vi "16BitsTo4ByteFloat.vi"(9 "Array":bool[](array[boolean]), 10 "Array 2":bool[](array[boolean]), 11 "Sign":bool) -> (1 "Mantissa 2":dbl=1.4518749713897705 format="%.8f", 2 "Numeric":sgl, 3 "Exponent":i32=6)   [LabVIEW 2014]
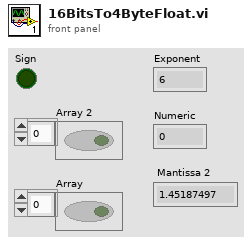
[diagram p1: front panel]
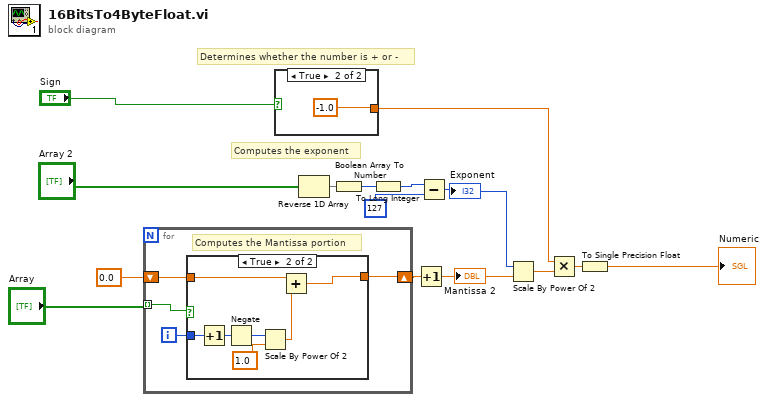
[diagram p0: block diagram]
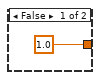
[diagram p2: hidden frame]
diagram:
  # "Computes the exponent"
  # "Determines whether the number is + or -"
  n1 = for {
    tunnel: "Array" -> [w19] mode=indexing
    shift-right: [w16] -> w2
    shift-left: 0.0 -> [w17]
    i -> [w18]
    # "Computes the Mantissa portion"
    n2 = case shown="True" w19 {
      tunnel: w18 -> [_ w27]
      tunnel: w17 -> [w20 w23]
      tunnel: [w20 w21] -> w16
      frame False {
      }
      frame True {
        n3 = Increment(x=w27) -> (x+1=w26:i32)
        n4 = Negate(x=w26) -> (-x=w25:i32)
        n5 = Scale By Power Of 2(n=w25, x=1.0) -> (x*2^n=w22:dbl)
        n6 = Add(x=w23, y=w22) -> (x+y=w21:dbl)
      }
    }
  }
  n7 = case shown="True" "Sign" {
    tunnel: [1.0 -1.0] -> w8
    frame False {
    }
    frame True {
    }
  }
  n8 = Reverse 1D Array(array="Array 2") -> (reversed array=w6:bool[])
  n9 = Boolean Array To Number(Boolean array=w6) -> (number=w10:u32)
  n10 = To Long Integer(number=w10) -> (32bit integer=w11:i32)
  n11 = Increment(x=w2) -> (x+1=w4:dbl)
  "Mantissa 2" <- w4
  n12 = Subtract(x=w11, y=127) -> (x-y=w9:i32)
  "Exponent" <- w9
  n13 = Scale By Power Of 2(n=w9, x=w4) -> (x*2^n=w5:dbl)
  n14 = Multiply(x=w8, y=w5) -> (x*y=w7:dbl)
  n15 = To Single Precision Float(number=w7) -> (single precision float=→"Numeric":sgl)
